vi "UBMExtract.vi"() -> ()   [LabVIEW 2022 SP3]
uses:
  <vilib>/Utility/file.llb/Write Delimited Spreadsheet (string).vi
panel:
  in  "Array 2":dbl[](array[numeric])
  in  "Save":bool
  in  "file path (dialog if empty)":path
  in  "Array 4":string[](array[string])=["Title (Dr. etc.) : ", "Full Name (first last) : ", "Are you self-nominating (i.e, speaking)\\? If space becomes limited, self-nominating speakers will have preference.: ", "Title of talk: ", "Self nomination description limited to 150 words (will not be published).: ", "Job Title: ", "Institution/Company: ", "Address:", "Email: ", "Mobile number: ", "Work Number: ", "Please let us know if you have any special requirements e.g. mobility, sight, diet etc.:", "Conference fees include accommodation for 3 nights (23, 24 and 25 September), all meals (3 breakfasts, 3 lunches, 3 dinners and coffee breaks), social events and the shuttle bus. Please indicate which of the following applies to you. Note that rates change after June 1.: ", "I would also like to book a place for an accompanying person (\\$650 includes accommodation for 23, 24 and 25 September, all conference meals, social events attendance and shuttle bus.: ", "Arrival - A shuttle bus is organized from New York City to Interlaken Inn. Would you like to book a place on this bus\\?: ", "Departure - A shuttle bus is organized from Interlaken Inn to New York City. Would you like to book a place on this bus\\?: ", "Please choose one of the following payment options - please note that if you are paying online you will have to submit this form first, then click the online payment link.: ", "I have read and agree to the Terms and Conditions of this event.: ", "I certify that payment for my attendance at UBM 2018 is being provided from my affiliated institution/business entity as indicated on the registration form. (No personally funded registrations are possible.): "]
  out "Array":string[](array[string])
  in  "String":string
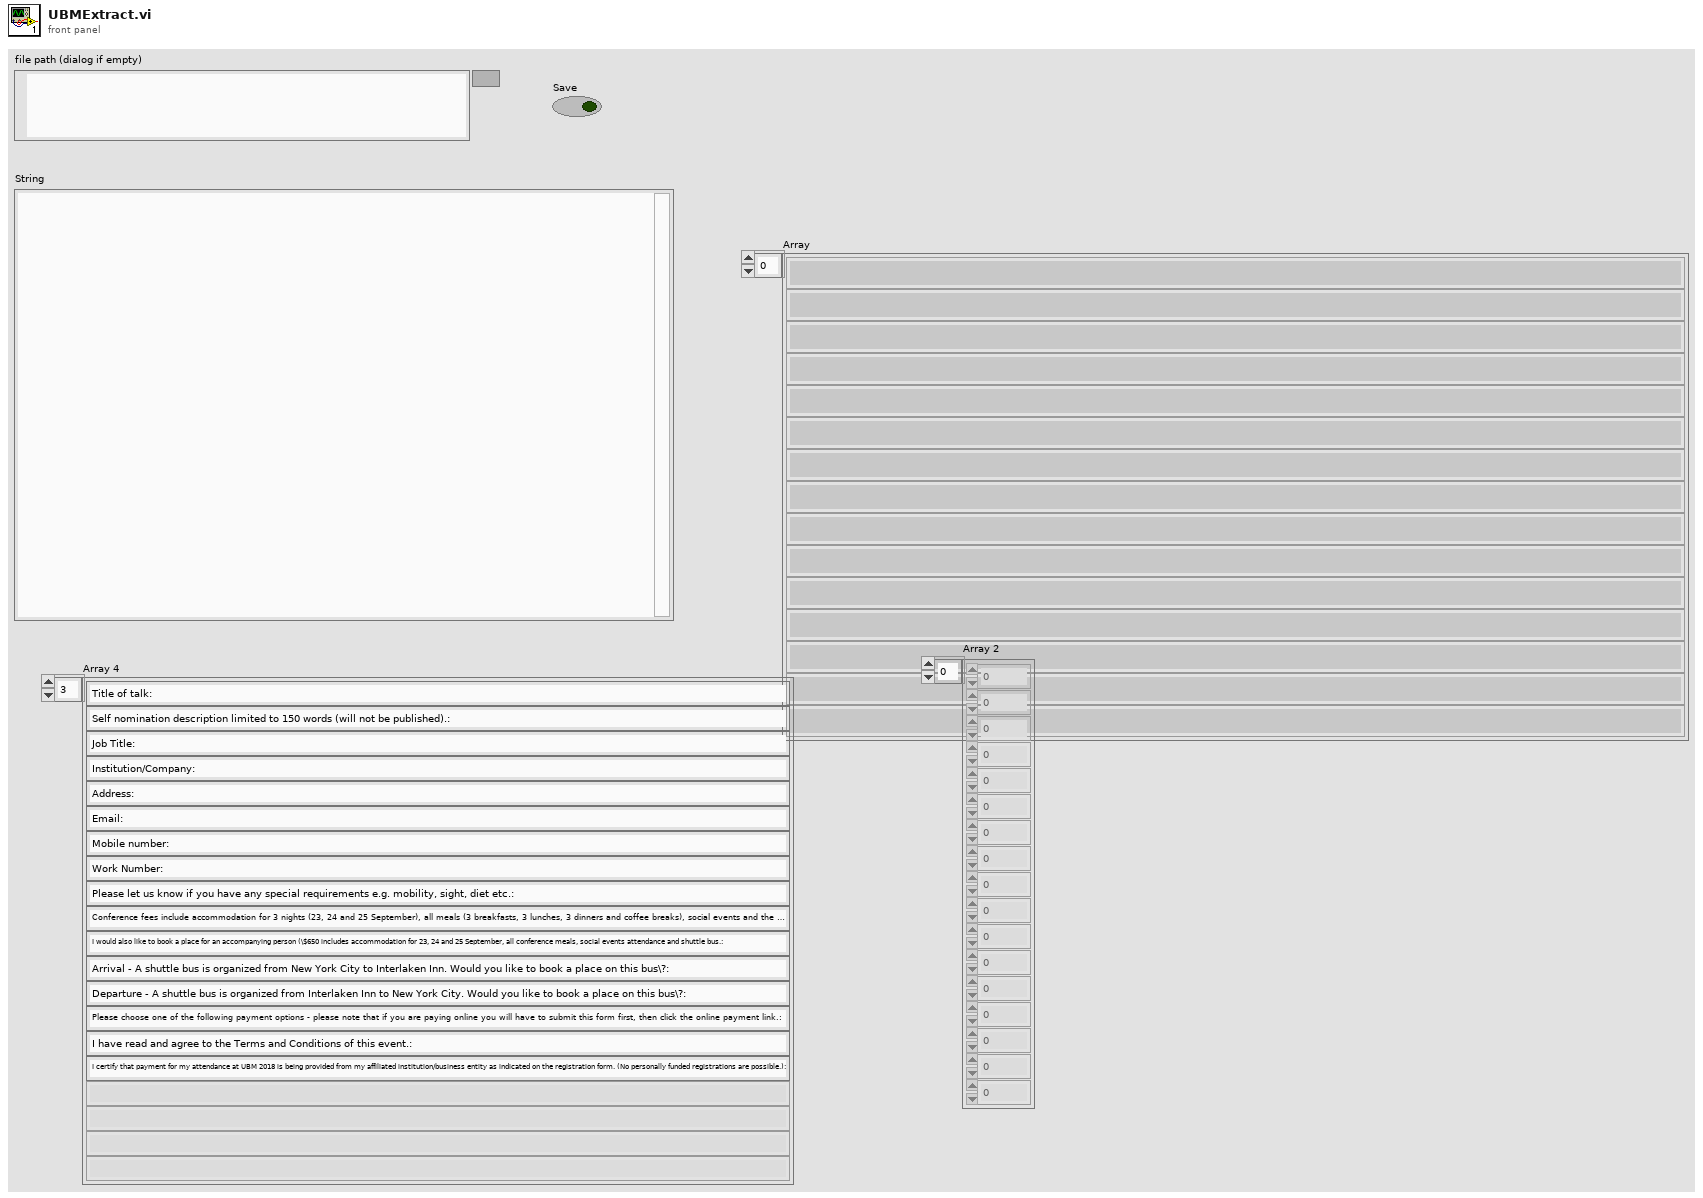
[diagram p1: front panel]
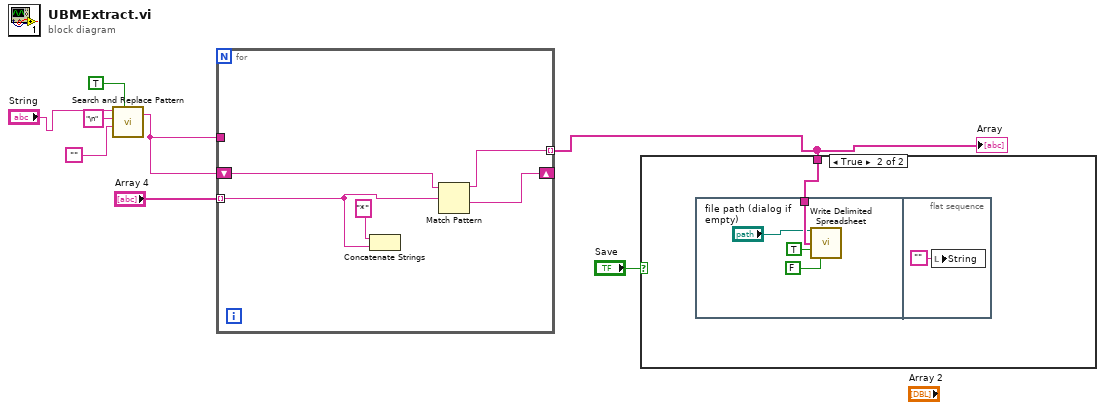
[diagram p0: block diagram]
diagram:
  n1 = call <vilib>:"Search and Replace Pattern.vi"("string"="String", "regular expression (\"\")"="\n" ("regular expression (\"\")"), "replace string (\"\")"="", "replace all? (F)"=TRUE) -> ("result string"=w4:string)  [unwired: 1 in, 1 out]
  n2 = for {
    shift-right: [w11] -> _
    shift-left: w4 -> [w12]
    tunnel: [w13] -> w1 mode=indexing
    tunnel: "Array 4" -> [w9] mode=indexing
    tunnel: w4 -> [_]
    n3 = Concatenate Strings("*", w9) -> ()  [unwired: 1 out]
    n4 = Match Pattern(string=w12, regular expression=w9) -> (before substring=w13:string, after substring=w11:string)  [unwired: 1 in, 2 out]
  }
  "Array" <- w1
  n5 = case shown="True" "Save" {
    tunnel: w1 -> [_ w14]
    frame False {
    }
    frame True {
      n6 = flat-sequence {
        tunnel: w14 -> [w18]
        frame #0 {
          n7 = call-poly <vilib>:"Write Delimited Spreadsheet.vi"("file path (dialog if empty)"="file path (dialog if empty)", "1D data"=w18, "append to file? (new file:F)"=TRUE, "transpose? (no:F)"=FALSE) -> ()  [unwired: 10 in, 2 out]
        }
        frame #1 {
          n8 = local write "String"("") -> ()
        }
      }
    }
  }
